vi "1D Array of VArrays to MultiD Array.vi"(8 "error in (no error)":errorcluster, 9 "Element Type":variant, 10 "Array of VArrays":variant[](array[variant]), 11 "Deserializer in":refnum<class "JSON Deserializer.lvclass">) -> (0 "error out":errorcluster, 2 "MultiD Array":variant, 3 "Deserializer out":refnum<class "JSON Deserializer.lvclass">)   [LabVIEW 2020, in "JKI JSON Serialization.lvlib" / "JSON Deserializer.lvclass"]
uses:
  JSON Deserializer.lvclass
  <userlib>/_OpenG.lib/lvdata/lvdata.llb/openg_variant.lvlib
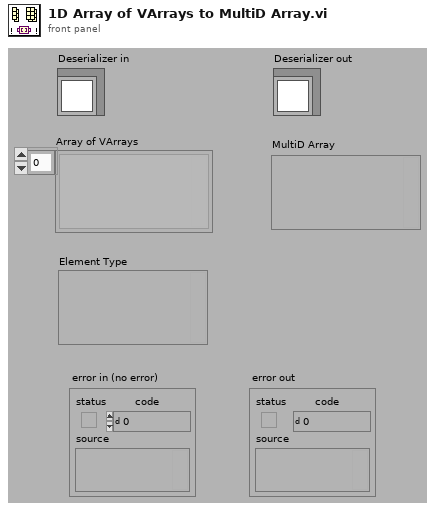
[diagram p1: front panel]
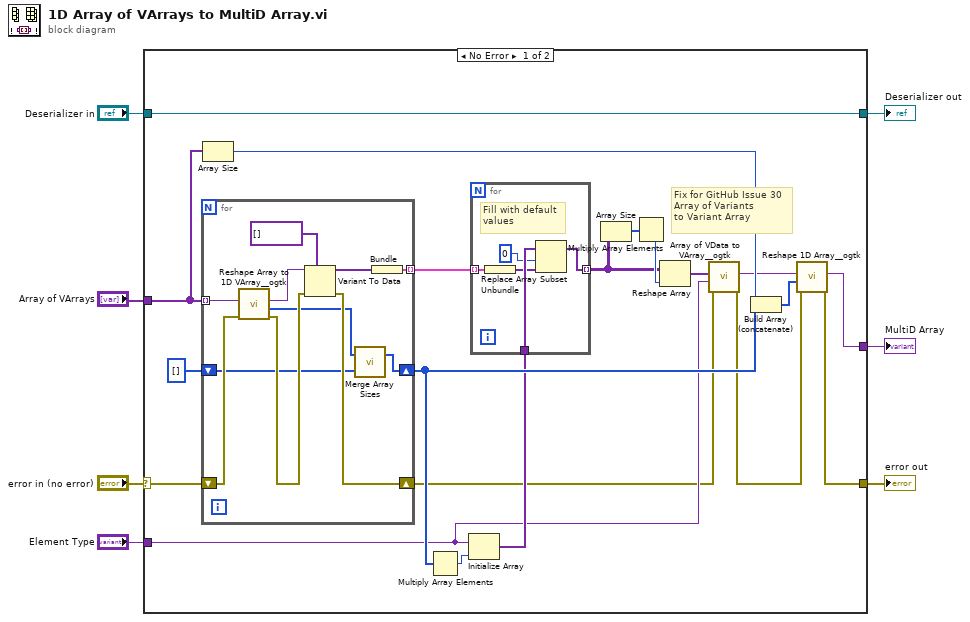
[diagram p0: block diagram]
diagram:
  n1 = case shown="No Error" "error in (no error)" {
    selector: "error in (no error)" -> [w27 w45]
    tunnel: [w23 w45] -> w7
    tunnel: [w20 _] -> w4
    tunnel: "Array of VArrays" -> [w26 _]
    tunnel: "Element Type" -> [w10 _]
    tunnel: "Deserializer in" -> [w13 w44]
    tunnel: [w13 w44] -> w1
    frame No Error {
      # "Fix for GitHub Issue 30\nArray of Variants\nto Variant Array"
      n2 = for {
        tunnel: w26 -> [w43] mode=indexing
        shift-right: [w39] -> w9
        shift-left: w27 -> [w42]
        tunnel: [w33] -> w18 mode=indexing
        shift-right: [w35] -> w16
        shift-left: i32[] [] -> [w36]
        n3 = call <userlib>:"Reshape Array to 1D VArray__ogtk.vi"("error in (no error)"=w42, "MultiD Array"=w43) -> ("error out"=w40:errorcluster, "Size(s)"=w34:u32[], "1D VArray"=w41:variant)  [unwired: 7 in]
        n4 = Variant To Data(error in=w40, type=variant[] [], Variant=w41) -> (data=w37:variant[], error out=w39:errorcluster)
        n5 = call "Merge Array Sizes.vi"("Sizes 2"=w36, "Sizes"=w34) -> ("Sizes out"=w35:i32[])  [unwired: 1 in]
        n6 = Bundle(w37) -> (w33:cluster{variant[]})  [unwired: 1 in]
      }
      n7 = Array Size(array=w26) -> (size(s)=w22:i32)
      n8 = Multiply Array Elements(1:w16) -> (0:w15:i32)
      n9 = Initialize Array(w10, w15) -> (w14:variant[])
      n10 = for {
        tunnel: w18 -> [w32] mode=indexing
        tunnel: [w31] -> w17 mode=indexing
        tunnel: w14 -> [w30]
        # "Fill with default\nvalues"
        n11 = Unbundle(w32) -> (w29:variant[])
        n12 = Replace Array Subset(array=w30, new element=w29, index=0) -> (w31:variant[])
      }
      n13 = Array Size(array=w17) -> (size(s)=w25:i32[])
      n14 = Multiply Array Elements(1:w25) -> (0:w24:i32)
      n15 = Reshape Array(w17, w24) -> (w12:variant[])
      n16 = call <userlib>:"Array of VData to VArray__ogtk.vi"("error in (no error)"=w9, "Element Type (when empty)"=w10, "1D Array of VData"=w12) -> ("error out"=w8:errorcluster, "VArray"=w11:variant)  [unwired: 7 in]
      n17 = Build Array (concatenate)(w22, w16) -> (w21:i32[])
      n18 = call <userlib>:"Reshape 1D Array__ogtk.vi"("error in (no error)"=w8, "Size(s)"=w21, "1D Array"=w11) -> ("error out"=w23:errorcluster, "Reshaped VArray"=w20:variant)  [unwired: 7 in]
    }
    frame Error {
    }
  }
  "error out" <- w7
  "MultiD Array" <- w4
  "Deserializer out" <- w1
